vi "Main.vi"(11 "Module Admin":refnum<class "Delacor_lib_QMH_Module Admin.lvclass">) -> ()   [LabVIEW 2026, in "CML UI.lvlib"]
doc: "This template is based off of the Queued Message Handler design pattern and the Queued Message Handler project template that ships with LabVIEW.\n\nThe main difference is that the queue is private to this module and communication between modules is performed via Broadcast and Request events.\n\nRequest events are wrapped in public API methods and are handled in the Event Handling Loop (EHL) of this VI. Any module can register for Broadcast events sent by this module. The EHL generates messages based on user interface actions.\n\nThe Message Handling Loop (MHL) processes messages generated by the EHL, or by other messages. The messages are string values, so new messages can be added easily to the Message Cases case structure in the MHL. Each message cluster can also provide an optional value for Message Data, which is a variant that can be converted to whatever message-specific data is required.\n_____\nBased on DQMH Project Template 4.0.0.47.\n_____\nBased on DQMH Dev Tools: Project Template 7.1.2.1547."
uses:
  CML UI.lvlib
  <vilib>/Delacor/Delacor QMH/Libraries/Module Admin_class/Delacor_lib_QMH_Module Admin.lvclass
  Module Data--cluster.ctl
  Stop Argument--cluster.ctl
  <vilib>/Delacor/Delacor QMH/Libraries/Message Queue_class/Delacor_lib_QMH_Message Queue.lvclass/Delacor_lib_QMH_Message Queue.ctl
  <vilib>/Delacor/Delacor QMH/Libraries/Module Admin_class/Delacor_lib_QMH_Module Admin.lvclass/Delacor_lib_QMH_Module Admin.ctl
  <vilib>/Delacor/Delacor QMH/Libraries/Message Queue_class/Delacor_lib_QMH_Enqueue Message (Single).vi
  <vilib>/Delacor/Delacor QMH/Libraries/Module Admin_class/Delacor_lib_QMH_Get External Launch.vi
  <vilib>/Delacor/Delacor QMH/Libraries/Message Queue_class/Delacor_lib_QMH_Message Queue.lvclass
  Settings Editor/Settings Editor.lvlib
  Acquisition/Acquisition.lvlib
  Logger/Logger.lvlib
panel:
  in  "About DQMH":bool
  out "Logger Running?":bool
  out "Settings Editor Running?":bool
  out "Acquisition Running?":bool
  out "Data":waveform(dbl)[](graph)
  out "Calibrated?":bool
  in  "Calibrate":bool
  in  "Settings":bool
  in  "Start":bool
  in  "Stop":bool
  out "error out":errorcluster
  out "Status":string
  out "version":string
  # "Continuous Measurement Data Logger"
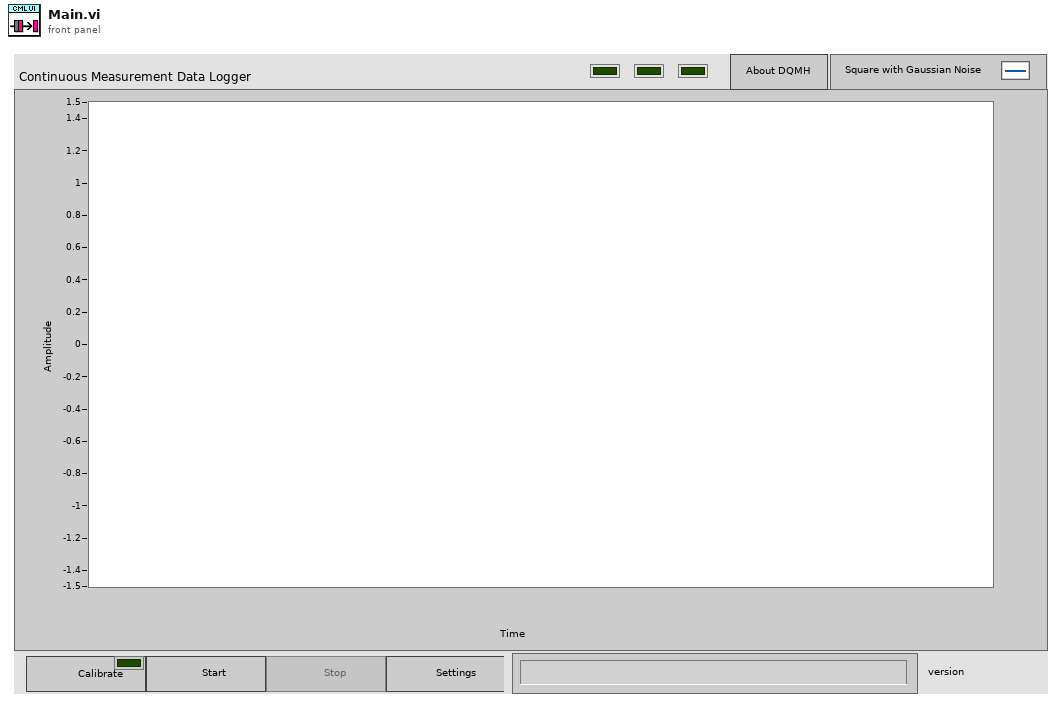
[diagram p1: front panel]
types:
  T1 = typedef "CML UI.lvlib/Request Events--cluster.ctl" = cluster{"Stop Module":refnum<user-event>, "Show Panel":refnum<user-event>, "Hide Panel":refnum<user-event>, "Get Module Execution Status":refnum<user-event>, "Show Diagram":refnum<user-event>}
  T2 = typedef "Settings Editor.lvlib/Broadcast Events--cluster.ctl" = cluster{"Module Did Init":refnum<user-event>, "Status Updated":refnum<user-event>, "Error Reported":refnum<user-event>, "Module Did Stop":refnum<user-event>, "Update Module Execution Status":refnum<user-event>, "Application Settings Updated":refnum<user-event>}
  T3 = typedef "Acquisition.lvlib/Broadcast Events--cluster.ctl" = cluster{"Module Did Init":refnum<user-event>, "Status Updated":refnum<user-event>, "Error Reported":refnum<user-event>, "Module Did Stop":refnum<user-event>, "Update Module Execution Status":refnum<user-event>, "Acquisition Started":refnum<user-event>, "Acquisition Stopped":refnum<user-event>, "Data Updated":refnum<user-event>, "Device Calibrated":refnum<user-event>}
  T4 = typedef "Logger.lvlib/Broadcast Events--cluster.ctl" = cluster{"Module Did Init":refnum<user-event>, "Status Updated":refnum<user-event>, "Error Reported":refnum<user-event>, "Module Did Stop":refnum<user-event>, "Update Module Execution Status":refnum<user-event>, "Logging Stopped":refnum<user-event>, "File Initialized":refnum<user-event>}
  T5 = typedef "CML UI.lvlib/Module Data--cluster.ctl" = cluster{"Status":string, "Start Ref":refnum<vi>, "Settings Ref":refnum<vi>, "Stop Ref":refnum<vi>, "Status Ref":refnum<vi>, "Data Ref":refnum<vi>}
  T6 = enum32{"invalid lock state", "Not Locked", "Locked (No Password)", "Password-protected"}
  T7 = typedef "CML UI.lvlib/Stop Argument--cluster.ctl" = cluster{"Origin":string, "Exit via Stop Module Req?":bool, "Wait for Module to stop?":bool}
  T8 = enum32{"Invalid", "Standard", "Closed", "Hidden", "Minimized", "Maximized"}
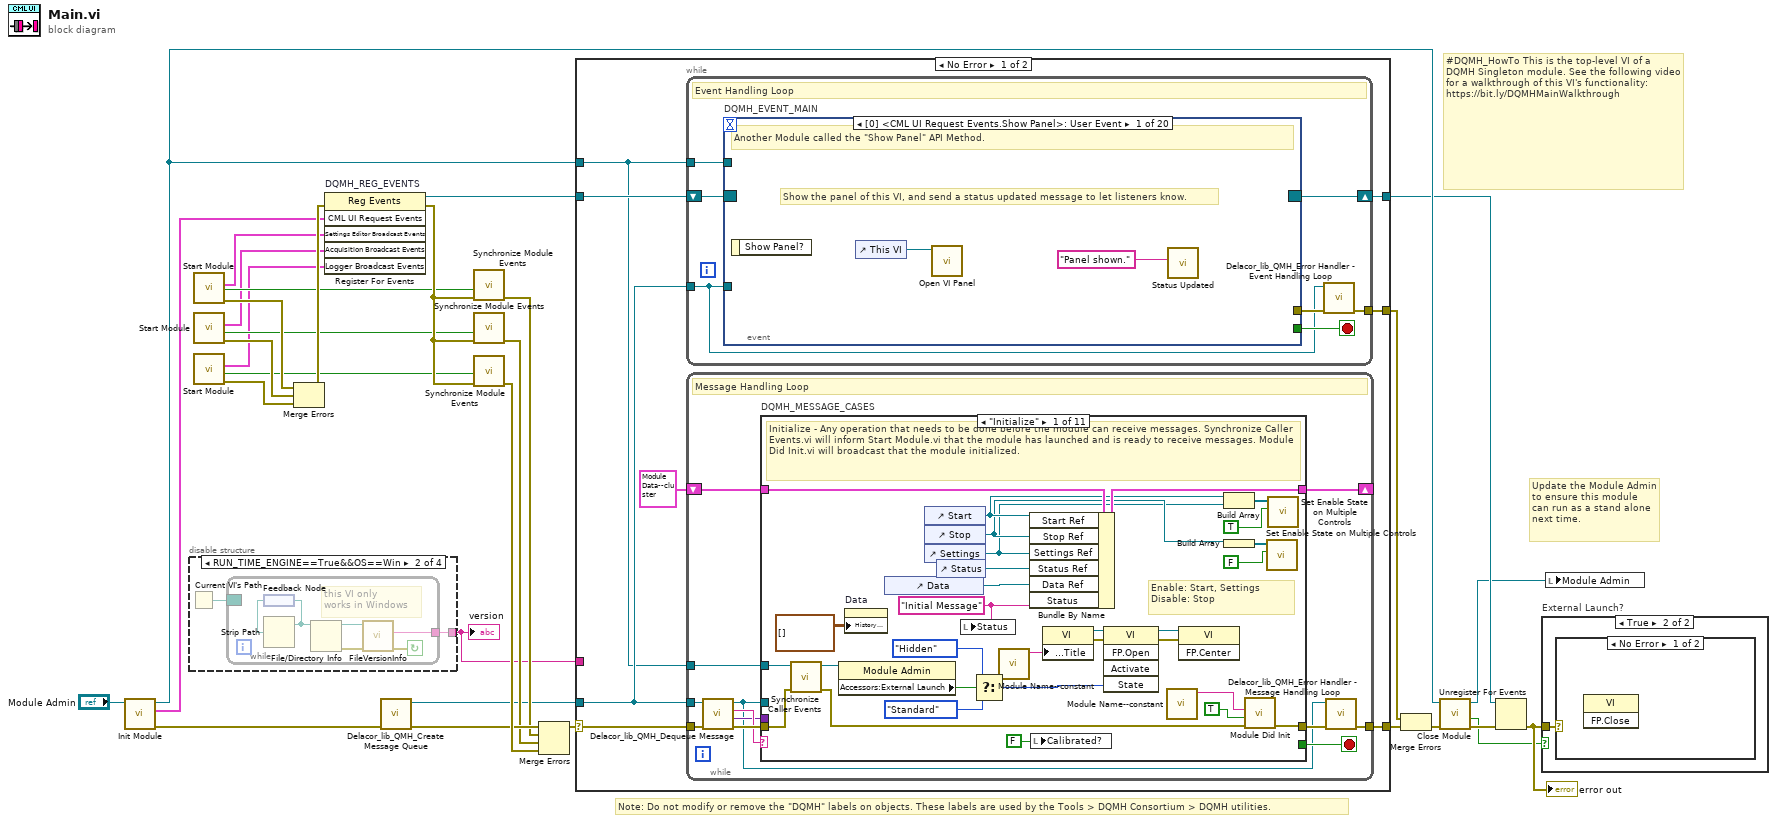
[diagram p0: block diagram]
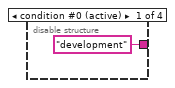
[diagram p2: hidden frame]
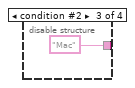
[diagram p3: hidden frame]
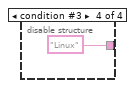
[diagram p4: hidden frame]
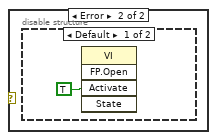
[diagram p6: hidden frame]
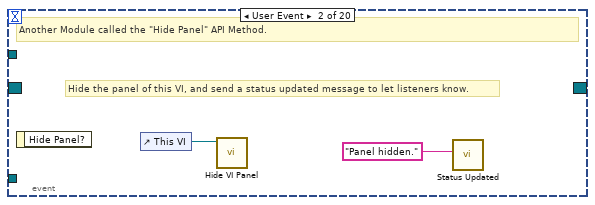
[diagram p8: hidden frame]
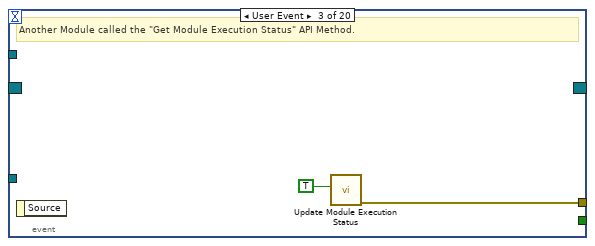
[diagram p9: hidden frame]
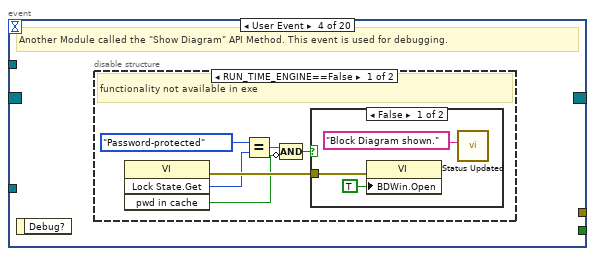
[diagram p10: hidden frame]
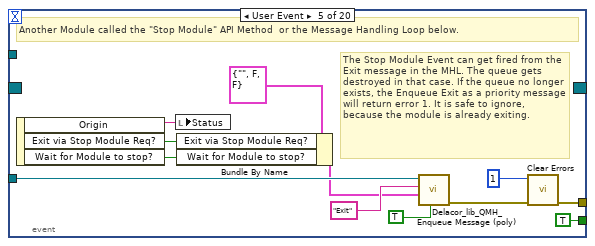
[diagram p13: hidden frame]
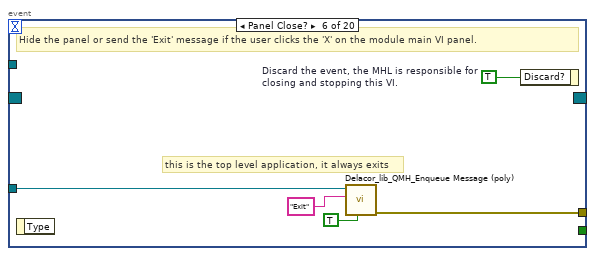
[diagram p14: hidden frame]
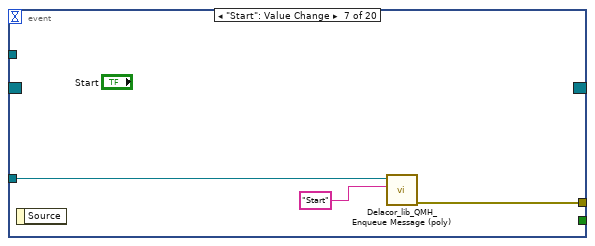
[diagram p15: hidden frame]
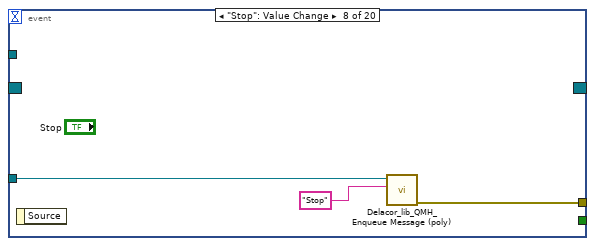
[diagram p16: hidden frame]
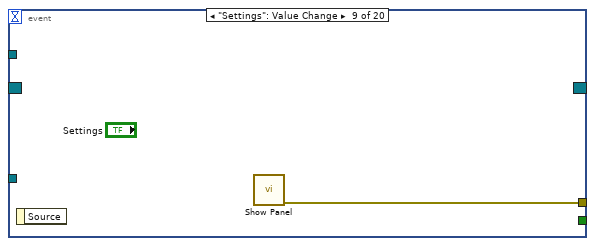
[diagram p17: hidden frame]
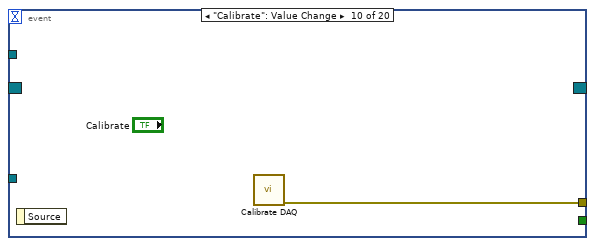
[diagram p18: hidden frame]
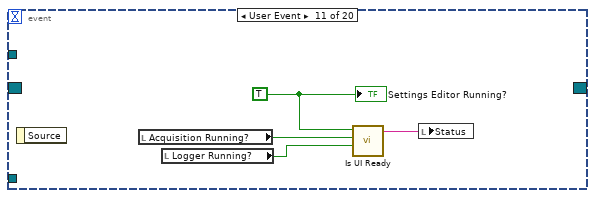
[diagram p19: hidden frame]
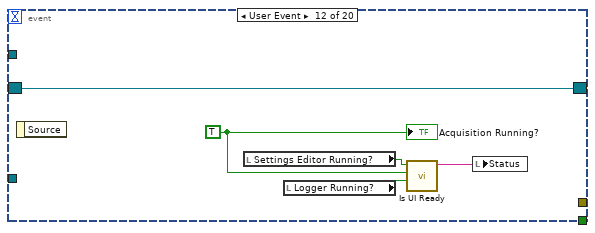
[diagram p20: hidden frame]
diagram:
  # "#DQMH_HowTo This is the top-level VI of a DQMH Singleton module. See the following video for a walkthrough of this VI's functionality: https://bit.ly/DQMHMainWalkthrough"
  # "Note: Do not modify or remove the \"DQMH\" labels on objects. These labels are used by the Tools > DQMH Consortium > DQMH utilities."
  # "Update the Module Admin to ensure this module can run as a stand alone next time."
  n1 = call "Init Module.vi"("Singleton Module Admin in"="Module Admin") -> ("error out"=w29:errorcluster, "CML UI Request Events"=w12:T1, "Singleton Module Admin out"=w15:refnum<class "Delacor_lib_QMH_Module Admin.lvclass">)  [unwired: 8 in]
  n2 = disable-structure "Conditional Disable Structure" shown="RUN_TIME_ENGINE==True&&OS==Win" {
    disable-tunnel: ["development" w33 "Mac" "Linux"] -> w1
    frame condition #0 (active) {
    }
    frame condition #1 {
      n3 = Current VI's Path() -> (path=w34:path)
      n4 = while {
        border: w34 -> [_]
        tunnel: [w35] -> w33
        stop <- w39 continue-if-true
        # "this VI only \nworks in Windows"
        n5 = feedback #1() -> (w38:path)
        n6 = Strip Path(path=w38) -> (stripped path=w37:path)  [unwired: 1 out]
        n7 = feedback-in #1(w37) -> ()
        n8 = File/Directory Info(path=w37) -> (path out=w36:path, error out=w40:errorcluster)  [unwired: 1 in, 5 out]
        n9 = call <vilib>:"FileVersionInfo.vi"("error in (no error)"=w40, "Application Path in"=w36) -> ("error out"=w39:errorcluster, "File Version Info"=w35:string)  [unwired: 6 in, 2 out]
      }
    }
    frame condition #2 {
    }
    frame condition #3 {
    }
  }
  "version" <- w1
  n10 = call "Start Module.vi"() -> ("error out"=w20:errorcluster, "Wait for Event Sync?"=w7:bool, "Settings Editor Broadcast Events"=w6:T2)  [unwired: 7 in, 2 out]
  n11 = call "Start Module.vi"() -> ("error out"=w19:errorcluster, "Wait for Event Sync?"=w4:bool, "Acquisition Broadcast Events"=w5:T3)  [unwired: 7 in, 2 out]
  n12 = call "Start Module.vi"() -> ("error out"=w18:errorcluster, "Wait for Event Sync?"=w2:bool, "Logger Broadcast Events"=w3:T4)  [unwired: 7 in, 2 out]
  n13 = Merge Errors(w20, w19, w18) -> (w17:errorcluster)
  n14 = register-events "DQMH_REG_EVENTS"(error in=w17, w12, w6, w5, w3) -> (reference out=w13:refnum<event-registration>, error out=w16:errorcluster)  [unwired: 1 in]
  n15 = call <vilib>:"Delacor_lib_QMH_Create Message Queue.vi"("error in"=w29) -> ("error out"=w24:errorcluster, "Message Queue"=w11:refnum<class "Delacor_lib_QMH_Message Queue.lvclass">)  [unwired: 9 in]
  n16 = call "Synchronize Module Events.vi"("error in"=w16, "Wait for Event Sync?"=w7) -> ("error out"=w22:errorcluster)  [unwired: 9 in]
  n17 = call "Synchronize Module Events.vi"("error in"=w16, "Wait for Event Sync?"=w4) -> ("error out"=w21:errorcluster)  [unwired: 9 in]
  n18 = call "Synchronize Module Events.vi"("error in"=w16, "Wait for Event Sync?"=w2) -> ("error out"=w31:errorcluster)  [unwired: 9 in]
  n19 = Merge Errors(w24, w22, w21, w31) -> (w23:errorcluster)
  n20 = case shown="No Error" w23 {
    selector: w23 -> [w48 w256]
    tunnel: [w50 w255] -> w30
    tunnel: [w47 w254] -> w14
    tunnel: w13 -> [w45 w254]
    tunnel: w11 -> [w44 w247]
    tunnel: [w49 _] -> w27
    tunnel: w15 -> [w43 w250]
    tunnel: w1 -> [_ _]
    frame No Error {
      n21 = while {
        tunnel: w44 -> [w51]
        shift-right: [w54] -> w47
        shift-left: w45 -> [w55]
        tunnel: [w56] -> w49
        tunnel: w43 -> [w52]
        stop <- w53 stop-if-true
        # "Event Handling Loop"
        n22 = event "DQMH_EVENT_MAIN" shown="[0] <CML UI Request Events.Show Panel>: User Event" {
          selector: w55 -> [_ _ _ _ _ _ _ _ _ _ _ w106 _ _ _ _ _ _ _ _]
          dyn-events: [_ _ _ _ _ _ _ _ _ _ _ w106 _ _ _ _ _ _ _ _] -> w54
          timeout: _ -> [_ _ _ _ _ _ _ _ _ _ _ _ _ _ _ _ _ _ _ _]
          tunnel: [_ _ _ _ TRUE ("Discard?") _ _ _ _ _ _ _ _ _ _ _ _ _ _ _] -> w53
          tunnel: w51 -> [_ _ _ _ w80 w87 w90 w93 _ _ _ _ _ _ _ w118 w120 _ _ _]
          tunnel: [_ _ w63 _ w83 w89 w92 w95 w96 w97 _ _ _ _ w116 _ _ _ _ w123] -> w57
          tunnel: w52 -> [_ _ _ _ _ _ _ _ _ _ _ _ _ _ _ _ _ _ _ _]
          event User Event {
            # "Show the panel of this VI, and send a status updated message to let listeners know."
            # "Another Module called the \"Show Panel\" API Method."
            n23 = event-data() -> ()  [unwired: 1 in, 1 out]
            n24 = control-ref of="This VI"() -> (w59:refnum<vi>)
            n25 = call "Open VI Panel.vi"("VI"=w59) -> ()  [unwired: 10 in, 1 out]
            n26 = call "Status Updated.vi"("Status"="Panel shown." ("format string")) -> ()  [unwired: 10 in, 1 out]
          }
          event User Event {
            # "Hide the panel of this VI, and send a status updated message to let listeners know."
            # "Another Module called the \"Hide Panel\" API Method."
            n27 = event-data() -> ()  [unwired: 1 in, 1 out]
            n28 = control-ref of="This VI"() -> (w61:refnum<vi>)
            n29 = call "Hide VI Panel.vi"("VI"=w61) -> ()  [unwired: 10 in, 1 out]
            n30 = call "Status Updated.vi"("Status"="Panel hidden." ("format string")) -> ()  [unwired: 10 in, 1 out]
          }
          event User Event {
            # "Another Module called the \"Get Module Execution Status\" API Method."
            n31 = event-data() -> ()  [unwired: 1 in, 1 out]
            n32 = call "Update Module Execution Status.vi"("Running?"=TRUE) -> ("error out"=w63:errorcluster)  [unwired: 10 in]
          }
          event User Event {
            # "Another Module called the \"Show Diagram\" API Method. This event is used for debugging."
            n33 = event-data() -> ()  [unwired: 1 in, 1 out]
            n34 = disable-structure shown="RUN_TIME_ENGINE==False" {
              frame condition #0 (active) {
                # "functionality not available in exe"
                n35 = invoke on="Invoke Node" class="VI" method="Lock State.Get"() -> (error out=w69:errorcluster, "Get Lock State"=w68:T6, "pwd in cache"=w65:bool)  [unwired: 4 in, 1 out]
                n36 = Equal?(x=T6."Password-protected", y=w68) -> (x = y?=w66:bool)
                n37 = Compound Arithmetic op=AND(w66, invert w65) -> (w64:bool)
                n38 = case shown="False" w64 {
                  tunnel: w69 -> [w72 _]
                  frame False {
                    n39 = property on="Property Node" class="VI"(error in=w72, "BDWin.Open"=TRUE ("Block Diagram Window:Open")) -> ()  [unwired: 1 in, 2 out]
                    n40 = call "Status Updated.vi"("Status"="Block Diagram shown." ("format string")) -> ()  [unwired: 10 in, 1 out]
                  }
                  frame True {
                    # "Password-protected VI, and the password is not in the cache. Do not show the diagram."
                  }
                }
              }
              frame condition #1 {
              }
            }
          }
          event User Event {
            # "The Stop Module Event can get fired from the Exit message in the MHL. The queue gets destroyed in that case. If the queue no longer exists, the Enqueue Exit as a priority message will return error 1. It is safe to ignore, because the module is already exiting."
            # "Another Module called the \"Stop Module\" API Method  or the Message Handling Loop below."
            n41 = event-data() -> ("Origin"=w79:string, "Exit via Stop Module Req?"=w75:bool, "Wait for Module to stop?"=w74:bool)  [unwired: 1 in]
            n42 = local write "Status"(w79) -> ()
            n43 = Bundle By Name(cluster=T7 {"Origin"="", "Exit via Stop Module Req?"=FALSE, "Wait for Module to stop?"=FALSE} ("Stop Argument"), "Exit via Stop Module Req?"=w75, "Wait for Module to stop?"=w74) -> (w73:T7)
            n44 = call-poly <vilib>:"Delacor_lib_QMH_Enqueue Message (poly).vi"("Priority Message? (F)"=TRUE, "Message Data"=w73, "Message"="Exit", "Message Queue in"=w80) -> ("error out"=w84:errorcluster)  [unwired: 6 in, 1 out]
            n45 = call <vilib>:"Clear Errors.vi"("error in (no error)"=w84, "specific error code to clear (0: all)"=1) -> ("error out"=w83:errorcluster)  [unwired: 4 in, 1 out]
          }
          event Panel Close? {
            w88 = TRUE  # Discard the event, the MHL is responsible for closing and stopping this VI.
            # "this is the top level application, it always exits"
            # "Hide the panel or send the 'Exit' message if the user clicks the 'X' on the module main VI panel."
            n46 = event-data() -> ()  [unwired: 1 in, 1 out]
            n47 = call-poly <vilib>:"Delacor_lib_QMH_Enqueue Message (poly).vi"("Priority Message? (F)"=TRUE, "Message"="Exit", "Message Queue in"=w87) -> ("error out"=w89:errorcluster)  [unwired: 7 in, 1 out]
            n48 = event-data ("Event Filter Node")("Discard?"=w88) -> ()  [unwired: 1 in, 1 out]
          }
          event "Start": Value Change {
            n49 = event-data() -> ()  [unwired: 1 in, 1 out]
            n50 = call-poly <vilib>:"Delacor_lib_QMH_Enqueue Message (poly).vi"("Message"="Start", "Message Queue in"=w90) -> ("error out"=w92:errorcluster)  [unwired: 8 in, 1 out]
          }
          event "Stop": Value Change {
            n51 = event-data() -> ()  [unwired: 1 in, 1 out]
            n52 = call-poly <vilib>:"Delacor_lib_QMH_Enqueue Message (poly).vi"("Message"="Stop", "Message Queue in"=w93) -> ("error out"=w95:errorcluster)  [unwired: 8 in, 1 out]
          }
          event "Settings": Value Change {
            n53 = event-data() -> ()  [unwired: 1 in, 1 out]
            n54 = call "Show Panel.vi"() -> ("error out"=w96:errorcluster)  [unwired: 11 in]
          }
          event "Calibrate": Value Change {
            n55 = event-data() -> ()  [unwired: 1 in, 1 out]
            n56 = call "Calibrate DAQ.vi"() -> ("error out"=w97:errorcluster)  [unwired: 11 in]
          }
          event User Event {
            w99 = TRUE ("Settings Editor Running?")
            n57 = event-data() -> ()  [unwired: 1 in, 1 out]
            n58 = local read "Acquisition Running?"() -> (w101:bool)
            n59 = local read "Logger Running?"() -> (w100:bool)
            n60 = call "Is UI Ready.vi"("Logger Running?"=w100, "Acquisition Running?"=w101, "Settings Editor Running?"=w99) -> ("Status"=w98:string)  [unwired: 8 in]
            n61 = local write "Status"(w98) -> ()
            "Settings Editor Running?" <- w99
          }
          event User Event {
            w104 = TRUE ("Acquisition Running?")
            n62 = event-data() -> ()  [unwired: 1 in, 1 out]
            n63 = local read "Settings Editor Running?"() -> (w103:bool)
            n64 = local read "Logger Running?"() -> (w102:bool)
            n65 = call "Is UI Ready.vi"("Logger Running?"=w102, "Acquisition Running?"=w104, "Settings Editor Running?"=w103) -> ("Status"=w105:string)  [unwired: 8 in]
            n66 = local write "Status"(w105) -> ()
            "Acquisition Running?" <- w104
          }
          event User Event {
            w109 = TRUE ("Logger Running?")
            n67 = event-data() -> ()  [unwired: 1 in, 1 out]
            n68 = local read "Settings Editor Running?"() -> (w108:bool)
            n69 = local read "Acquisition Running?"() -> (w107:bool)
            n70 = call "Is UI Ready.vi"("Logger Running?"=w109, "Acquisition Running?"=w107, "Settings Editor Running?"=w108) -> ("Status"=w110:string)  [unwired: 8 in]
            n71 = local write "Status"(w110) -> ()
            "Logger Running?" <- w109
          }
          event User Event {
            n72 = event-data() -> ("Status"=w111:string)  [unwired: 1 in]
            "Status" <- w111
            n73 = call "Status Updated.vi"("Status"=w111) -> ()  [unwired: 10 in, 1 out]
          }
          event User Event {
            n74 = event-data() -> ("Error"=w116:errorcluster, "Module Name"=w114:string)  [unwired: 1 in]
            n75 = Unbundle By Name(w116) -> ("code"=w115:i32)
            n76 = Format Into String(format string="Error %d at %s", w115, w114) -> (resulting string=w113:string)  [unwired: 2 in, 1 out]
            n77 = local write "Status"(w113) -> ()
          }
          event User Event {
            n78 = event-data() -> ()  [unwired: 1 in, 1 out]
            n79 = call-poly <vilib>:"Delacor_lib_QMH_Enqueue Message (poly).vi"("Message"="Acquisition Started Interlocks", "Message Queue in"=w118) -> ()  [unwired: 8 in, 2 out]
          }
          event User Event {
            n80 = event-data() -> ()  [unwired: 1 in, 1 out]
            n81 = call-poly <vilib>:"Delacor_lib_QMH_Enqueue Message (poly).vi"("Message"="Acquisition Stopped Interlocks", "Message Queue in"=w120) -> ()  [unwired: 8 in, 2 out]
          }
          event User Event {
            n82 = event-data() -> ("Graph Data"=→"Data":waveform(dbl)[])  [unwired: 1 in]
          }
          event User Event {
            n83 = event-data() -> ()  [unwired: 1 in, 1 out]
            "Calibrated?" <- TRUE ("Calibrated?")
          }
          event "About DQMH": Value Change {
            # "Display the About DQMH box"
            n84 = event-data() -> ()  [unwired: 1 in, 1 out]
            n85 = call <vilib>:"DQMH_About Box.vi"() -> ("error out"=w123:errorcluster)  [unwired: 11 in]
          }
        }
        n86 = call-dynamic "Delacor_lib_QMH_Error Handler - Event Handling Loop.vi"("error in"=w57, "Message Queue in"=w51) -> ("dup error in"=w56:errorcluster)  [unwired: 8 in, 1 out]
      }
      n87 = while {
        tunnel: w44 -> [w126]
        shift-right: [w130] -> _
        shift-left: T5 {"Status"="", "Start Ref"=refnum, "Settings Ref"=refnum, "Stop Ref"=refnum, "Status Ref"=refnum, "Data Ref"=refnum} ("Data Cluster") -> [w131]
        tunnel: w48 -> [w134]
        tunnel: [w132] -> w50
        tunnel: w43 -> [w124]
        stop <- w129 stop-if-true
        # "Message Handling Loop"
        n88 = call-dynamic "Delacor_lib_QMH_Dequeue Message.vi"("error in"=w134, "Message Queue in"=w126) -> ("error out"=w133:errorcluster, "Message Data"=w127:variant, "Message"=w128:string, "Message Queue out"=w125:refnum<class "Delacor_lib_QMH_Message Queue.lvclass">)  [unwired: 6 in]
        n89 = case "DQMH_MESSAGE_CASES" shown="\"Initialize\"" w128 {
          selector: w128 -> [_ _ _ _ _ _ _ _ _ _ w242]
          tunnel: w125 -> [_ _ _ _ _ _ _ _ w201 w226 _]
          tunnel: w133 -> [w163 w167 w170 w180 w183 w193 w196 w198 w209 w234 w245]
          tunnel: [w161 w167 w169 w180 w182 w193 w195 w198 w205 w227 w246] -> w135
          tunnel: w131 -> [w152 w166 w168 w172 w181 w185 w194 w197 w203 w225 w243]
          tunnel: [w144 w166 w168 w172 w181 w185 w194 w197 w203 w225 w243] -> w130
          tunnel: [_ _ _ _ _ _ _ _ _ w224 _] -> w129
          tunnel: w127 -> [_ _ _ _ _ _ _ _ w202 w223 _]
          tunnel: w124 -> [w153 _ _ _ _ _ _ _ w200 w218 _]
          frame "Initialize" {
            w147 = "Initial Message" ("Initial Message")
            # "Enable: Start, Settings\nDisable: Stop"
            # "Initialize - Any operation that needs to be done before the module can receive messages. Synchronize Caller Events.vi will inform Start Module.vi that the module has launched and is ready to receive messages. Module Did Init.vi will broadcast that the module initialized."
            n90 = call "Synchronize Caller Events.vi"("error in"=w163, "Singleton Module Admin in"=w153) -> ("error out"=w162:errorcluster, "Singleton Module Admin out"=w149:refnum<class "Delacor_lib_QMH_Module Admin.lvclass">)  [unwired: 8 in]
            n91 = property on="Property Node" class="Module Admin"(reference=w149) -> ("Accessors:External Launch"=w157:bool)  [unwired: 1 in, 2 out]
            n92 = property on="Data" class="WFChart (strict)"("History Data"=waveform(dbl)[][] []) -> ()  [unwired: 2 in, 2 out]
            n93 = control-ref of="Data"() -> (w145:refnum<vi>)
            n94 = control-ref of="Start"() -> (w138:refnum<vi>)
            n95 = control-ref of="Stop"() -> (w137:refnum<vi>)
            n96 = control-ref of="Settings"() -> (w136:refnum<vi>)
            n97 = control-ref of="Status"() -> (w146:refnum<vi>)
            n98 = local write "Status"(w147) -> ()
            n99 = Select(t=T8."Hidden" ("State"), s=w157, f=T8."Standard" ("State")) -> (s? t:f=w154:T8)
            n100 = call "Module Name--constant.vi"() -> ("Module Name"=w160:string)  [unwired: 11 in]
            n101 = Bundle By Name(cluster=w152, "Start Ref"=w138, "Stop Ref"=w137, "Settings Ref"=w136, "Status Ref"=w146, "Data Ref"=w145, "Status"=w147) -> (w144:T5)
            n102 = local write "Calibrated?"(FALSE ("Calibrated?")) -> ()
            n103 = property on="Property Node" class="VI"("Front Panel.Title"=w160) -> (reference out=w159:refnum<vi>, error out=w165:errorcluster)  [unwired: 2 in]
            n104 = invoke on="Invoke Node" class="VI" method="FP.Open"(reference=w159, error in=w165, "State"=w154) -> (reference out=w158:refnum<vi>, error out=w164:errorcluster)  [unwired: 2 in, 3 out]
            n105 = call "Module Name--constant.vi"() -> ("Module Name"=w150:string)  [unwired: 11 in]
            n106 = invoke on="Invoke Node" class="VI" method="FP.Center"(reference=w158, error in=w164) -> ()  [unwired: 1 in, 3 out]
            n107 = Build Array(w138, w136) -> (w143:refnum<vi>[])
            n108 = Build Array(w137) -> (w141:refnum<vi>[])
            n109 = call "Module Did Init.vi"("error in"=w162, "Initialized?"=TRUE, "Origin"=w150) -> ("error out"=w161:errorcluster)  [unwired: 8 in]
            n110 = call "Set Enable State on Multiple Controls.vi"("Enable?"=FALSE, "Controls"=w141) -> ()  [unwired: 10 in]
            n111 = call "Set Enable State on Multiple Controls.vi"("Enable?"=TRUE, "Controls"=w143) -> ()  [unwired: 10 in]
          }
          frame "---Module Specific---" {
            # "Separator -- The following cases handle messages specific to this Module."
          }
          frame "Start" {
            # "End user pressed Start button. Need to request for Acquisition to start acquiring and for Logger to start logging."
            n112 = call "Initialize File.vi"("error in"=w170) -> ("error out"=w171:errorcluster)  [unwired: 8 in, 2 out]
            n113 = call "Start Acquiring.vi"("error in"=w171) -> ("error out"=w169:errorcluster)  [unwired: 8 in, 2 out]
          }
          frame "Acquisition Started Interlocks" {
            # "Enable: Stop\nDisable: Start, Settings"
            n114 = Unbundle By Name(w172) -> ("Stop Ref"=w179:refnum<vi>, "Start Ref"=w174:refnum<vi>, "Settings Ref"=w173:refnum<vi>)
            n115 = Build Array(w179) -> (w178:refnum<vi>[])
            n116 = Build Array(w174, w173) -> (w175:refnum<vi>[])
            n117 = call "Set Enable State on Multiple Controls.vi"("Enable?"=TRUE, "Controls"=w178) -> ()  [unwired: 10 in]
            n118 = call "Set Enable State on Multiple Controls.vi"("Enable?"=FALSE, "Controls"=w175) -> ()  [unwired: 10 in]
          }
          frame "Stop" {
            # "End user pressed Stop button. Need to request for Acquisition to stop acquiring and for Logger to stop logging."
            n119 = call "Stop Acquiring.vi"("error in"=w183) -> ("error out"=w184:errorcluster)  [unwired: 10 in]
            n120 = call "Stop Logging.vi"("error in"=w184) -> ("error out"=w182:errorcluster)  [unwired: 10 in]
          }
          frame "Acquisition Stopped Interlocks" {
            # "Enable: Start, Settings\nDisable: Stop"
            n121 = Unbundle By Name(w185) -> ("Stop Ref"=w190:refnum<vi>, "Start Ref"=w189:refnum<vi>, "Settings Ref"=w188:refnum<vi>)
            n122 = Build Array(w190) -> (w192:refnum<vi>[])
            n123 = Build Array(w189, w188) -> (w187:refnum<vi>[])
            n124 = call "Set Enable State on Multiple Controls.vi"("Enable?"=FALSE, "Controls"=w192) -> ()  [unwired: 10 in]
            n125 = call "Set Enable State on Multiple Controls.vi"("Enable?"=TRUE, "Controls"=w187) -> ()  [unwired: 10 in]
          }
          frame "---Copy This Frame---" {
            # "Duplicate this frame when creating new messages.  Change this comment in the duplicated frame to describe this message."
            n126 = Merge Errors(w196) -> (w195:errorcluster)
          }
          frame "---Exit and Error Handling---" {
            # "Separator - The following cases handle errors and exit messages."
          }
          frame "Error" {
            # "Error - Check the error message data and respond accordingly. This message is sent by the \"Error Handler\" VIs at the end of each loop in this application."
            n127 = property on="Property Node" class="Module Admin"(reference=w200) -> ("Accessors:External Launch"=w199:bool)  [unwired: 1 in, 2 out]
            n128 = Variant To Data(error in=w209, type=errorcluster {"status"=FALSE, "code"=0, "source"=""} ("error constant"), Variant=w202) -> (data=w204:errorcluster, error out=w207:errorcluster)
            n129 = local write "error out"(w204) -> ()
            n130 = call "Error Reported.vi"("Error"=w204) -> ()  [unwired: 10 in, 1 out]
            n131 = case shown="False" w199 {
              tunnel: [w214 _] -> w206
              tunnel: w201 -> [w212 _]
              tunnel: w204 -> [w213 _]
              frame False {
                n132 = disable-structure shown="Default" {
                  disable-tunnel: w213 -> [w215 _]
                  frame condition #0 (active) {
                    # "If the module is running standalone, then pop up an error dialog and call the \"Exit\" message."
                    n133 = call <vilib>:"Simple Error Handler.vi"("error in (no error)"=w215) -> ()  [unwired: 4 in, 5 out]
                  }
                  frame condition #1 {
                    # "To prevent the Simple Error Handler VI from being loaded (e.g. when deploying to a Real-Time target), add the Conditional Disable Symbol \"DQMH_Disable_SEH\" to your project and set it to TRUE."
                  }
                }
                n134 = call-poly <vilib>:"Delacor_lib_QMH_Enqueue Message (poly).vi"("Priority Message? (F)"=TRUE, "Message"="Exit", "Message Queue in"=w212) -> ("error out"=w214:errorcluster)  [unwired: 7 in, 1 out]
              }
              frame True {
                # "If the module was launched externally, calling the Error Reported broadcast VI is the only action performed by the \"Error\" message. The module's caller can then process the error appropriately."
              }
            }
            n135 = Merge Errors(w207, w206) -> (w205:errorcluster)
          }
          frame "Exit" {
            w217 = TRUE ("Wait for Module to Stop? (F)")
            w224 = TRUE  # Stop the VI
            # "DAQ and LOG modules use the settings editor. CML UI module waits for both modules to completely stop before stopping the settings editor."
            # "Release the message queue reference"
            # "Exit - Exit the application."
            n136 = Variant To Data(error in=w234, type=T7 {"Origin"="", "Exit via Stop Module Req?"=FALSE, "Wait for Module to stop?"=FALSE} ("Stop Argument"), Variant=w223) -> (data=w220:T7, error out=w231:errorcluster)
            n137 = call <vilib>:"Clear Errors.vi"("error in (no error)"=w231, "specific error code to clear (0: all)"=91 ("91: not all Exit messages will have an argument")) -> ("error out"=w233:errorcluster)  [unwired: 4 in, 1 out]
            n138 = control-ref of="This VI"() -> (w219:refnum<vi>)
            n139 = call "Module Name--constant.vi"() -> ("Module Name"=w216:string)  [unwired: 11 in]
            n140 = call "Handle Exit.vi"("Stop Argument"=w220, "Admin in"=w218, "VI reference"=w219) -> ("error out"=w230:errorcluster)  [unwired: 7 in, 1 out]
            n141 = call "Stop Module.vi"("Wait for Module to Stop? (F)"=w217, "Origin"=w216) -> ("error out"=w229:errorcluster)  [unwired: 9 in]
            n142 = call "Stop Module.vi"("Wait for Module to Stop? (F)"=w217, "Origin"=w216) -> ("error out"=w228:errorcluster)  [unwired: 9 in]
            n143 = call-dynamic "Delacor_lib_QMH_Release Message Queue.vi"("error in"=w233, "Message Queue"=w226) -> ("error out"=w232:errorcluster)  [unwired: 9 in]
            n144 = Merge Errors(w229, w228) -> (w235:errorcluster)
            n145 = Merge Errors(w232, w230) -> (w227:errorcluster)
            n146 = call <vilib>:"Clear Errors.vi"("error in (no error)"=w235) -> ("error out"=w236:errorcluster)  [unwired: 5 in, 1 out]
            n147 = call "Error Reported.vi"("Error"=w227) -> ()  [unwired: 10 in, 1 out]
            n148 = call "Stop Module.vi"("error in"=w236, "Wait for Module to Stop? (F)"=w217, "Origin"=w216) -> ()  [unwired: 8 in, 1 out]
          }
          frame Default {
            # "'Default' case only runs if there is a message that isn't defined in any of the other cases.  Output a programming error."
            n149 = call "Module Name--constant.vi"() -> ("Module Name"=w241:string)  [unwired: 11 in]
            n150 = Format Into String(format string="The invalid message string \"%s\" was received in the Message Handling Loop for module \"%s\".", w242, w241) -> (resulting string=w239:string)  [unwired: 2 in, 1 out]
            n151 = call <vilib>:"Error Cluster From Error Code.vi"("show call chain? (False)"=TRUE, "error message (\"\")"=w239, "error code (0)"=1) -> ("error out"=w244:errorcluster)  [unwired: 6 in]
            n152 = Merge Errors(w245, w244) -> (w246:errorcluster)
          }
        }
        n153 = call-dynamic "Delacor_lib_QMH_Error Handler - Message Handling Loop.vi"("error in"=w135, "Message Queue in"=w125) -> ("dup error in"=w132:errorcluster)  [unwired: 8 in, 1 out]
      }
    }
    frame Error {
      w249 = TRUE ("Wait for Module to Stop? (F)")
      # "Synchronize Caller Events.vi will inform Start Module.vi that the module has launched and will let the code calling Start Module.vi register for broadcasts and would permit the caller receive the broadcast that an error occurred at launch time."
      n154 = call-dynamic "Delacor_lib_QMH_Release Message Queue.vi"("error in"=w256, "Message Queue"=w247) -> ("error out"=w255:errorcluster)  [unwired: 9 in]
      n155 = call "Synchronize Caller Events.vi"("Singleton Module Admin in"=w250) -> ("error out"=w257:errorcluster)  [unwired: 9 in, 1 out]
      n156 = call "Module Name--constant.vi"() -> ("Module Name"=w253:string)  [unwired: 11 in]
      n157 = call "Module Name--constant.vi"() -> ("Module Name"=w248:string)  [unwired: 11 in]
      n158 = call "Stop Module.vi"("Wait for Module to Stop? (F)"=w249, "Origin"=w248) -> ()  [unwired: 9 in, 1 out]
      n159 = call "Stop Module.vi"("Wait for Module to Stop? (F)"=w249, "Origin"=w248) -> ()  [unwired: 9 in, 1 out]
      n160 = call "Stop Module.vi"("Wait for Module to Stop? (F)"=w249, "Origin"=w248) -> ()  [unwired: 9 in, 1 out]
      n161 = Format Into String(format string="An error occurred during initialization. %s is no longer running.", w253) -> (resulting string=w251:string)  [unwired: 2 in, 1 out]
      n162 = Merge Errors(w255, w257) -> (w258:errorcluster)
      n163 = call "Error Reported.vi"("Additional Information"=w251, "Error"=w258) -> ()  [unwired: 9 in, 1 out]
    }
  }
  n164 = Merge Errors(w27, w30) -> (w26:errorcluster)
  n165 = call "Close Module.vi"("error in"=w26, "Module Admin in"=w15) -> ("error out"=w28:errorcluster, "External Launch"=w8:bool, "Module Admin out"=w9:refnum<class "Delacor_lib_QMH_Module Admin.lvclass">)  [unwired: 7 in]
  n166 = Unregister For Events(event registration refnum=w14, error in=w28) -> (error out=w25:errorcluster)
  "error out" <- w25
  n167 = case "External Launch?" shown="True" w8 {
    tunnel: w25 -> [_ w259]
    frame False {
    }
    frame True {
      n168 = case shown="No Error" w259 {
        frame No Error {
          n169 = invoke on="Invoke Node" class="VI" method="FP.Close"() -> ()  [unwired: 3 in, 3 out]
        }
        frame Error {
          n170 = disable-structure shown="Default" {
            frame condition #0 (active) {
              n171 = invoke class="VI" method="FP.Open"("Activate"=TRUE ("Activate?")) -> ()  [unwired: 4 in, 5 out]
            }
            frame condition #1 {
              # "Don't show panel on error if running inside a built EXE."
            }
          }
        }
      }
    }
  }
  n172 = local write "Module Admin"(w9) -> ()
